vi "load images.vi"() -> ()   [LabVIEW 2016]
uses:
  <vilib>/picture/picture.llb/imagedata.ctl
panel:
  in  "apply offsets?":bool=TRUE
  out "image data":T1[](array[typedef])
  in  "Path":path
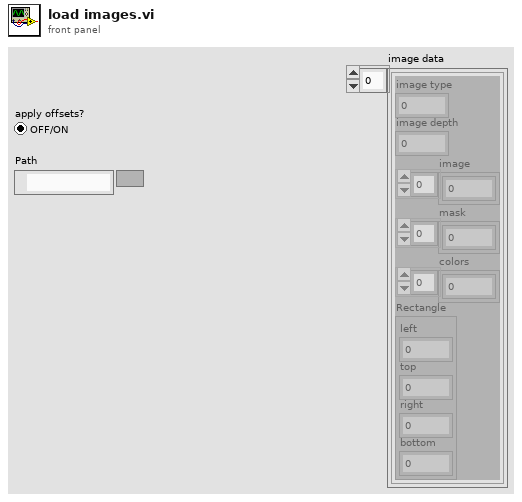
[diagram p1: front panel]
types:
  T1 = typedef "imagedata.ctl" = cluster{"image type":i32, "image depth":i32, "image":u8[], "mask":u8[], "colors":u32[], "Rectangle":cluster{"left":i16, "top":i16, "right":i16, "bottom":i16}}
  T2 = cluster{"left":i16, "top":i16, "right":i16, "bottom":i16}
  T3 = cluster{"left":i16, "top":i16, "right":i16, "bottom":i16}[]
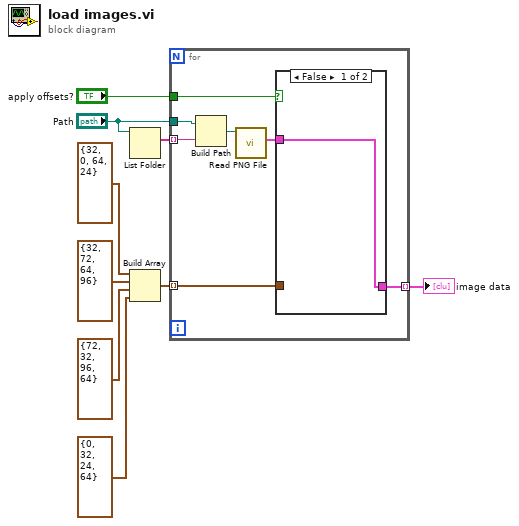
[diagram p0: block diagram]
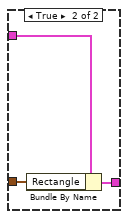
[diagram p2: hidden frame]
diagram:
  n1 = List Folder(path="Path") -> (filenames=w8:string[])  [unwired: 3 in, 3 out]
  n2 = Build Array(T2 {"left"=32, "top"=0, "right"=64, "bottom"=24} ("Rectangle"), T2 {"left"=32, "top"=72, "right"=64, "bottom"=96} ("Rectangle"), T2 {"left"=72, "top"=32, "right"=96, "bottom"=64} ("Rectangle"), T2 {"left"=0, "top"=32, "right"=24, "bottom"=64} ("Rectangle")) -> (w2:T3)
  n3 = for {
    tunnel: "Path" -> [w16]
    tunnel: w8 -> [w15] mode=indexing
    tunnel: [w12] -> w7 mode=indexing
    tunnel: w2 -> [w11] mode=indexing
    tunnel: "apply offsets?" -> [w10]
    n4 = Build Path(base path=w16, name or relative path=w15) -> (appended path=w14:path)
    n5 = call <vilib>:"Read PNG File.vi"("path to PNG file"=w14) -> ("image data"=w13:T1)  [unwired: 8 in, 2 out]
    n6 = case shown="False" w10 {
      tunnel: w13 -> [w17 w20]
      tunnel: [w17 w19] -> w12
      tunnel: w11 -> [_ w18]
      frame False {
      }
      frame True {
        n7 = Bundle By Name(cluster=w20, "Rectangle"=w18) -> (w19:T1)
      }
    }
  }
  "image data" <- w7
